vi "Done.vi"(8 "error in (no error)":errorcluster, 11 "State in":refnum<class "State.lvclass">) -> (0 "error out":errorcluster, 2 "Done?":bool, 3 "State out":refnum<class "State.lvclass">)   [LabVIEW 2019, in "23.lvlib" / "State.lvclass"]
uses:
  State.lvclass
  C:/Users/craig.walker/Documents/GitHub/lv2019-LRU-Cache/LRU Node/LRU Node.lvclass
  lv2019-LRU-Cache/LRU Node/LRU Node.lvclass/LRU Node.ctl
  State Key/State Key.lvclass/State Key.ctl
  lv2019-LRU-Cache/LRU Node/Read Key.vi
  State Key/State Key.lvclass
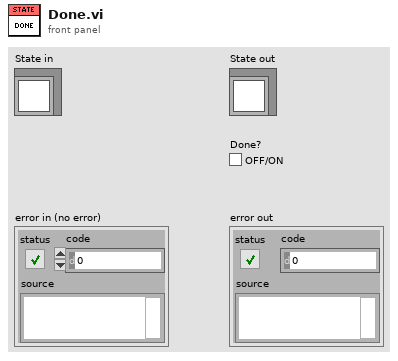
[diagram p1: front panel]
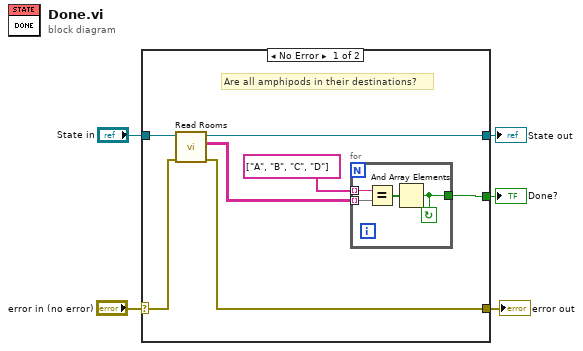
[diagram p0: block diagram]
diagram:
  n1 = case shown="No Error" "error in (no error)" {
    selector: "error in (no error)" -> [w7 w17]
    tunnel: "State in" -> [w10 w18]
    tunnel: [w9 w18] -> w4
    tunnel: [w12 _] -> w3
    tunnel: [w6 w17] -> w1
    frame No Error {
      # "Are all amphipods in their destinations?"
      n2 = call "Read Rooms.vi"("error in (no error)"=w7, "State in"=w10) -> ("error out"=w6:errorcluster, "Rooms"=w8:string[][], "State out"=w9:refnum<class "State.lvclass">)  [unwired: 7 in]
      n3 = for {
        tunnel: w8 -> [w14] mode=indexing
        tunnel: [w15] -> w12
        tunnel: string[] ["A", "B", "C", "D"] -> [w13] mode=indexing
        stop <- w15 continue-if-true
        n4 = Equal?(x=w13, y=w14) -> (x = y?=w16:bool[])
        n5 = And Array Elements(Boolean array=w16) -> (logical AND=w15:bool)
      }
    }
    frame Error {
    }
  }
  "Done?" <- w3
  "State out" <- w4
  "error out" <- w1
